vi "1SDI_Threshold_v00.vi"(6 "MaxMin":T1, 11 "Signals":T12={"PII In 1"={"Lock"=FALSE, "Hold"=FALSE, "P Gain"=0, "P BS"=0, "I Gain"=0, "I BS"=-10, "I2 G"=0, "I2 BS"=-26, "Scan Amp"=0, "Scan Off"=0, "Scan FS"=0, "SFS BS"=0, "I Max value"=10000, "I2 Max value"=10000, "Scope.Offset"=0, "Trigger Direction"=enum."either", "Scan-PII thresh"=0}, "PII In 2"={"Lock"=FALSE, "Hold"=FALSE, "P Gain"=0, "P BS"=0, "I Gain"=0, "I BS"=-10, "I2 G"=0, "I2 BS"=-26, "Scan Amp"=0, "Scan Off"=0, "Scan FS"=0, "SFS BS"=0, "I Max value"=10000, "I2 Max value"=10000, "Scope.Offset"=0, "Trigger Direction"=enum."either", "Scan-PII thresh"=0}, "PII In 3"={"Lock"=FALSE, "Hold"=FALSE, "P Gain"=0, "P BS"=0, "I Gain"=0, "I BS"=-10, "I2 G"=0, "I2 BS"=-26, "Scan Amp"=0, "Scan Off"=0, "Scan FS"=0, "SFS BS"=0, "I Max value"=10000, "I2 Max value"=10000, "Scope.Offset"=0, "Trigger Direction"=enum."either", "Scan-PII thresh"=0}, "Lock Thresh"={"EPR"=2, "HD A"=0, "HD B"=0}, "Re-Scan Thresh"={"EPR"=2, "HD A"=0, "HD B"=0}, "Safety First"={"lim reset"=FALSE, "no limit"=FALSE, "pos slew rate * dt"=0, "neg slew rate * dt"=-10, "Hold All"=FALSE, "Count(Ticks)"=4294967286}, "Graph Errors"={"EPR"=2, "HD A"=0, "HD B"=0}}) -> (3 "Control Graph Cluster":T8={"Control EPR"={"Lock"=FALSE, "Hold"=FALSE, "P Gain"=0, "P BS"=-5, "I Gain"=0, "I BS"=-10, "I2 G"=0, "I2 BS"=-26, "Scan Amp"=0, "Scan Off"=0, "Scan FS"=0, "SFS BS"=0, "I Max value"=10000, "I2 Max value"=10000, "Scope.Offset"=0, "Trigger Direction"=enum."either", "Scan-PII thresh"=0}, "Control HD A"={"Lock"=FALSE, "Hold"=FALSE, "P Gain"=0, "P BS"=-5, "I Gain"=0, "I BS"=-10, "I2 G"=0, "I2 BS"=-26, "Scan Amp"=0, "Scan Off"=0, "Scan FS"=0, "SFS BS"=0, "I Max value"=10000, "I2 Max value"=10000, "Scope.Offset"=0, "Trigger Direction"=enum."either", "Scan-PII thresh"=0}, "Control HD B"={"Lock"=FALSE, "Hold"=FALSE, "P Gain"=0, "P BS"=-5, "I Gain"=0, "I BS"=-10, "I2 G"=0, "I2 BS"=-26, "Scan Amp"=0, "Scan Off"=0, "Scan FS"=0, "SFS BS"=0, "I Max value"=10000, "I2 Max value"=10000, "Scope.Offset"=0, "Trigger Direction"=enum."either", "Scan-PII thresh"=0}, "Max"={"Max EPR"=0, "Max HD A"=0, "Max HD B"=0}, "Min"={"Min EPR"=0, "Min HD A"=0, "Min HD B"=0}, "Lock Threshold"={"EPR"=0, "HD A"=0, "HD B"=0}, "Re-Scan Threshold"={"EPR"=0, "HD A"=0, "HD B"=0}, "Lock Point?"={"EPR"=FALSE, "HD A"=FALSE, "HD B"=FALSE}, "Re-scan?"={"EPR"=FALSE, "HD A"=FALSE, "HD B"=FALSE}, "Lock pressed? (-1)"={"EPR"=FALSE, "HD A"=FALSE, "HD B"=FALSE}, "Cavity Errors"={"EPR"=0, "HD A"=0, "HD B"=0}, "State (-1)"={"EPR"=enum."Safe", "HD A"=enum."Safe", "HD B"=enum."Safe"}, "Safety First"={"lim reset"=FALSE, "no limit"=FALSE, "pos slew rate * dt"=0, "neg slew rate * dt"=0, "Hold All"=FALSE, "Count(Ticks)"=0}})   [LabVIEW 2013]
doc: "Determines if the relative phase of the two interfering beams are within a range determined by a user-defined threshold. The absolute value of the error signal is used as a monitor."
uses:
  Strict Type Defs/Signals 1SDI.ctl
  Strict Type Defs/PII individual.ctl
  Strict Type Defs/Lock Thresh 1SDI.ctl
  Strict Type Defs/Safety First.ctl
  Strict Type Defs/Error Signals 1SDI.ctl
  Strict Type Defs/1SDI Control Cluster.ctl
  Strict Type Defs/1SDI Max.ctl
  Strict Type Defs/1SDI Min.ctl
  Strict Type Defs/1SDI Lock Point.ctl
  Strict Type Defs/1SDI State.ctl
  Strict Type Defs/1SDI MaxMin.ctl
  Strict Type Defs/1SDI Reset MaxMin.ctl
panel:
  in  "Control Cavity Cluster":T8={"Control EPR"={"Lock"=FALSE, "Hold"=FALSE, "P Gain"=0, "P BS"=-5, "I Gain"=0, "I BS"=-10, "I2 G"=0, "I2 BS"=-26, "Scan Amp"=0, "Scan Off"=0, "Scan FS"=0, "SFS BS"=0, "I Max value"=10000, "I2 Max value"=10000, "Scope.Offset"=0, "Trigger Direction"=enum."either", "Scan-PII thresh"=0}, "Control HD A"={"Lock"=FALSE, "Hold"=FALSE, "P Gain"=0, "P BS"=-5, "I Gain"=0, "I BS"=-10, "I2 G"=0, "I2 BS"=-26, "Scan Amp"=0, "Scan Off"=0, "Scan FS"=0, "SFS BS"=0, "I Max value"=10000, "I2 Max value"=10000, "Scope.Offset"=0, "Trigger Direction"=enum."either", "Scan-PII thresh"=0}, "Control HD B"={"Lock"=FALSE, "Hold"=FALSE, "P Gain"=0, "P BS"=-5, "I Gain"=0, "I BS"=-10, "I2 G"=0, "I2 BS"=-26, "Scan Amp"=0, "Scan Off"=0, "Scan FS"=0, "SFS BS"=0, "I Max value"=10000, "I2 Max value"=10000, "Scope.Offset"=0, "Trigger Direction"=enum."either", "Scan-PII thresh"=0}, "Max"={"Max EPR"=0, "Max HD A"=0, "Max HD B"=0}, "Min"={"Min EPR"=0, "Min HD A"=0, "Min HD B"=0}, "Lock Threshold"={"EPR"=0, "HD A"=0, "HD B"=0}, "Re-Scan Threshold"={"EPR"=0, "HD A"=0, "HD B"=0}, "Lock Point?"={"EPR"=FALSE, "HD A"=FALSE, "HD B"=FALSE}, "Re-scan?"={"EPR"=FALSE, "HD A"=FALSE, "HD B"=FALSE}, "Lock pressed? (-1)"={"EPR"=FALSE, "HD A"=FALSE, "HD B"=FALSE}, "Cavity Errors"={"EPR"=0, "HD A"=0, "HD B"=0}, "State (-1)"={"EPR"=enum."Safe", "HD A"=enum."Safe", "HD B"=enum."Safe"}, "Safety First"={"lim reset"=FALSE, "no limit"=FALSE, "pos slew rate * dt"=0, "neg slew rate * dt"=0, "Hold All"=FALSE, "Count(Ticks)"=0}}
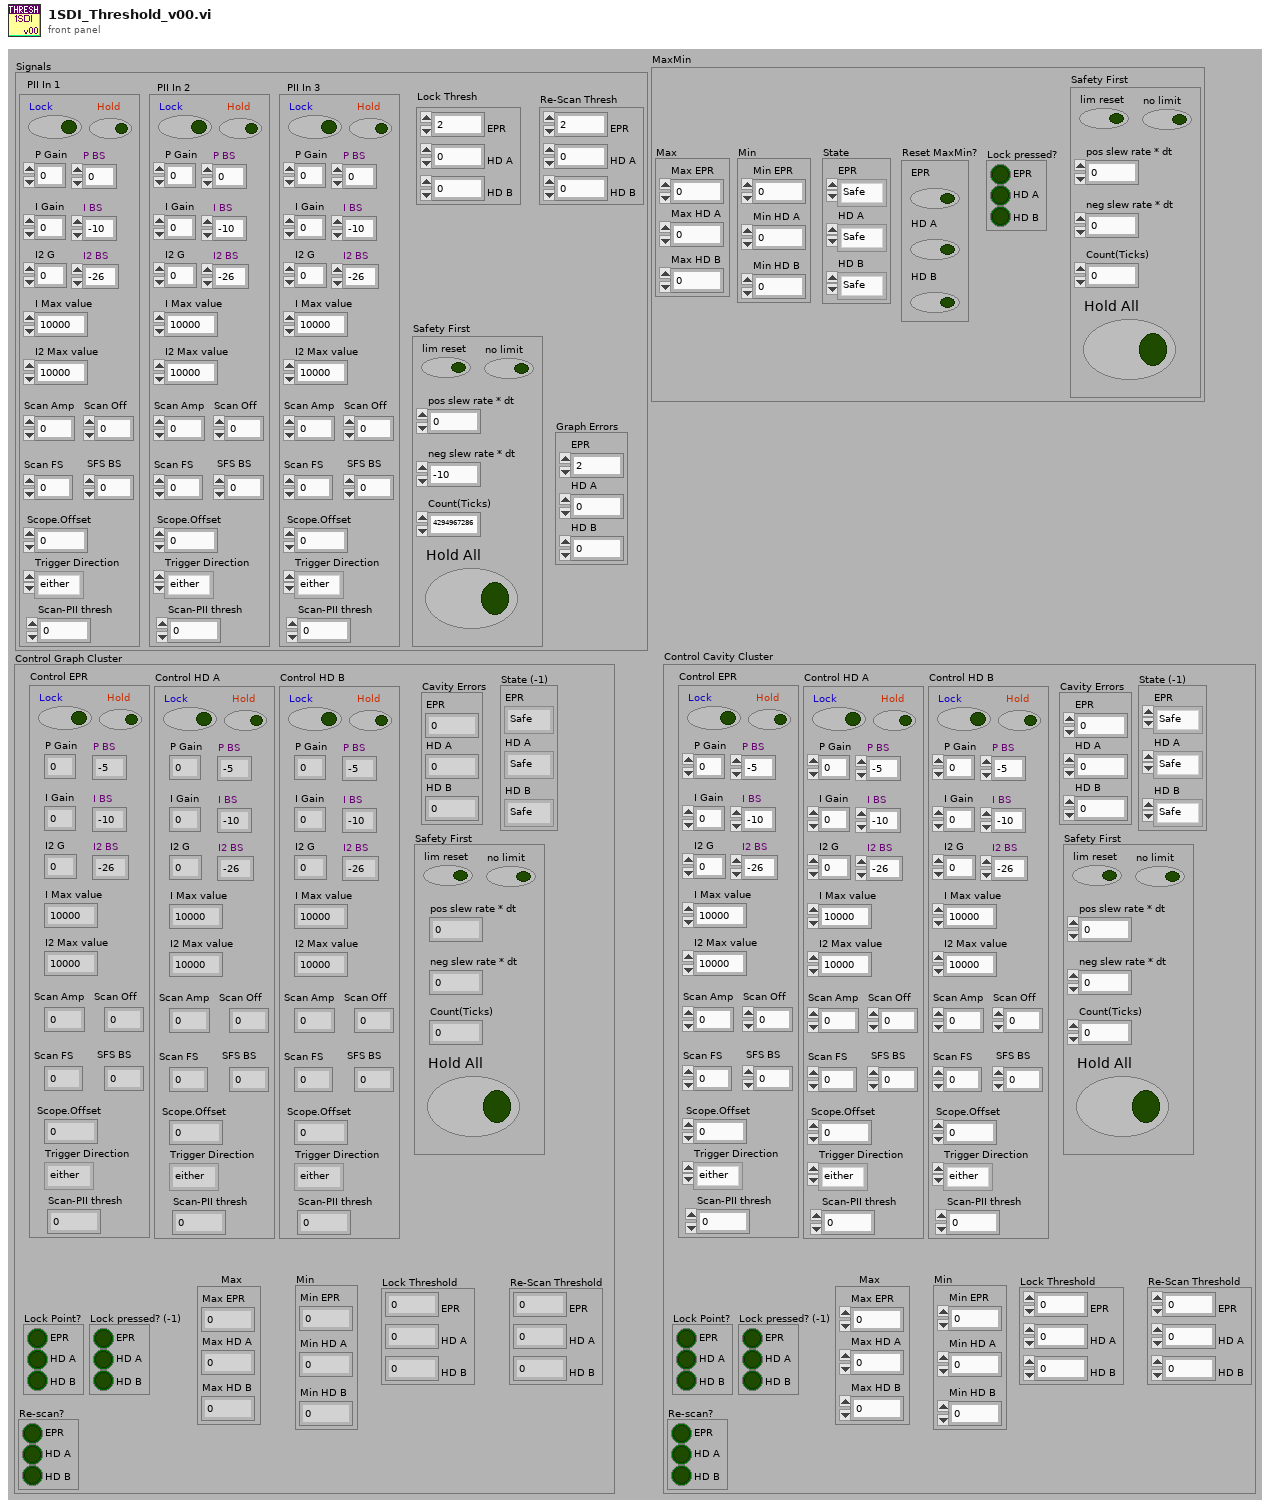
[diagram p1: front panel]
types:
  T1 = typedef "1SDI MaxMin.ctl" = cluster{"State":T2, "Reset MaxMin?":T3, "Max":T4, "Min":T5, "Lock pressed?":T6, "Safety First":T7}
  T2 = typedef "1SDI State.ctl" = cluster{"EPR":enum16{"Safe", "Hold", "Scan", "Lock"}, "HD A":enum16{"Safe", "Hold", "Scan", "Lock"}, "HD B":enum16{"Safe", "Hold", "Scan", "Lock"}}
  T3 = typedef "1SDI Reset MaxMin.ctl" = cluster{"EPR":bool, "HD A":bool, "HD B":bool}
  T4 = typedef "1SDI Max.ctl" = cluster{"Max EPR":i16, "Max HD A":i16, "Max HD B":i16}
  T5 = typedef "1SDI Min.ctl" = cluster{"Min EPR":i16, "Min HD A":i16, "Min HD B":i16}
  T6 = typedef "1SDI Lock Point.ctl" = cluster{"EPR":bool, "HD A":bool, "HD B":bool}
  T7 = typedef "Safety First.ctl" = cluster{"lim reset":bool, "no limit":bool, "pos slew rate * dt":i16, "neg slew rate * dt":i16, "Hold All":bool, "Count(Ticks)":u32}
  T8 = typedef "1SDI Control Cluster.ctl" = cluster{"Control EPR":T9, "Control HD A":T9, "Control HD B":T9, "Max":T4, "Min":T5, "Lock Threshold":T10, "Re-Scan Threshold":T10, "Lock Point?":T6, "Re-scan?":T6, "Lock pressed? (-1)":T6, "Cavity Errors":T11, "State (-1)":T2, "Safety First":T7}
  T9 = typedef "PII individual.ctl" = cluster{"Lock":bool, "Hold":bool, "P Gain":i32, "P BS":i16, "I Gain":i32, "I BS":i16, "I2 G":i32, "I2 BS":i16, "Scan Amp":i16, "Scan Off":i16, "Scan FS":u16, "SFS BS":i16, "I Max value":i32, "I2 Max value":i32, "Scope.Offset":i16, "Trigger Direction":enum8{"either", "minus-plus", "plus-minus"}, "Scan-PII thresh":i16}
  T10 = typedef "Lock Thresh 1SDI.ctl" = cluster{"EPR":i16, "HD A":i16, "HD B":i16}
  T11 = typedef "Error Signals 1SDI.ctl" = cluster{"EPR":i16, "HD A":i16, "HD B":i16}
  T12 = typedef "Signals 1SDI.ctl" = cluster{"PII In 1":T9, "PII In 2":T9, "PII In 3":T9, "Lock Thresh":T10, "Re-Scan Thresh":T10, "Safety First":T7, "Graph Errors":T11}
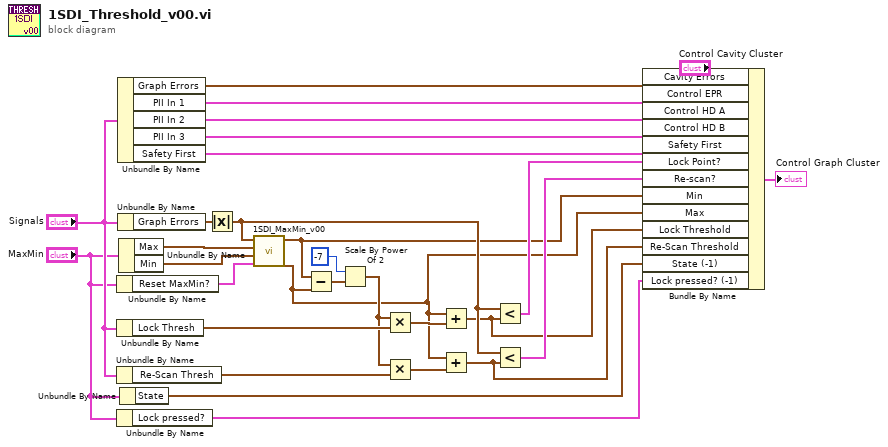
[diagram p0: block diagram]
diagram:
  n1 = Unbundle By Name("MaxMin") -> ("Reset MaxMin?"=w21:T3)
  n2 = Unbundle By Name("Signals") -> ("Lock Thresh"=w17:T10)
  n3 = Unbundle By Name("Signals") -> ("Re-Scan Thresh"=w23:T10)
  n4 = Unbundle By Name("MaxMin") -> ("Lock pressed?"=w1:T6)
  n5 = Unbundle By Name("Signals") -> ("Graph Errors"=w13:T11, "PII In 1"=w12:T9, "PII In 2"=w11:T9, "PII In 3"=w10:T9, "Safety First"=w9:T7)
  n6 = Unbundle By Name("Signals") -> ("Graph Errors"=w19:T11)
  n7 = Unbundle By Name("MaxMin") -> ("Max"=w29:T4, "Min"=w28:T5)
  n8 = Unbundle By Name("MaxMin") -> ("State"=w2:T2)
  n9 = Absolute Value(x=w19) -> (abs(x)=w18:T11)
  n10 = call "1SDI_MaxMin_v00.vi"("Reset MaxMin?"=w21, "Min (-1)"=w28, "Max (-1)"=w29, "Graph Errors"=w18) -> ("Max"=w5:T4, "Min"=w6:T5)  [unwired: 6 in]
  n11 = Subtract(x=w6, y=w5) -> (x-y=w26:T5)
  n12 = Scale By Power Of 2(n=-7, x=w26) -> (x*2^n=w16:T5)
  n13 = Multiply(x=w16, y=w17) -> (x*y=w25:T5)
  n14 = Multiply(x=w16, y=w23) -> (x*y=w24:T5)
  n15 = Add(x=w5, y=w25) -> (x+y=w4:T4)
  n16 = Add(x=w5, y=w24) -> (x+y=w3:T4)
  n17 = Less?(x=w18, y=w4) -> (x < y?=w8:cluster{bool, bool, bool})
  n18 = Less?(x=w18, y=w3) -> (x < y?=w7:cluster{bool, bool, bool})
  n19 = Bundle By Name(cluster="Control Cavity Cluster", "Cavity Errors"=w13, "Control EPR"=w12, "Control HD A"=w11, "Control HD B"=w10, "Safety First"=w9, "Lock Point?"=w8, "Re-scan?"=w7, "Min"=w6, "Max"=w5, "Lock Threshold"=w4, "Re-Scan Threshold"=w3, "State (-1)"=w2, "Lock pressed? (-1)"=w1) -> (→"Control Graph Cluster":T8)
